vi "Configure List Step.vi"(0 "VISA resource name":refnum<visa-resource-name>, 1 "List (0: Current List)":i32(ring) items=["Current List", "Voltage List"], 2 "Execution Times (1)":i32=1, 3 "Enable List Continuously (F: Disable)":bool, 5 "Channel (1)":string="1", 7 "List Step Setting (0: Automatically)":i32(ring) items=["Automatically", "Once"], 9 "Time Point (0 sec)":dbl[](array[numeric]) format="%#_3g", 11 "error in (no error)":errorcluster, 12 "Step Value List (0.001)":dbl[](array[numeric]) format="%#_3g", 13 "Begin Trigger Signal List Step (F: Disable)":bool[](array[boolean]), 14 "End Trigger Signal List Step (F: Disable)":bool[](array[boolean])) -> (4 "VISA resource name out":refnum<visa-resource-name>, 15 "error out":errorcluster)   [LabVIEW 2020, in "Keysight E36300 Series.lvlib"]
doc: "Configures the specified list value for each list step.\n\n<b>Notes: </b>\n(1)This VI is only available on the E36312A and E36313A models.\n(2)The list is up to 100 steps.\n(3)This VI overwrites previously programmed list."
uses:
  Keysight E36300 Series.lvlib
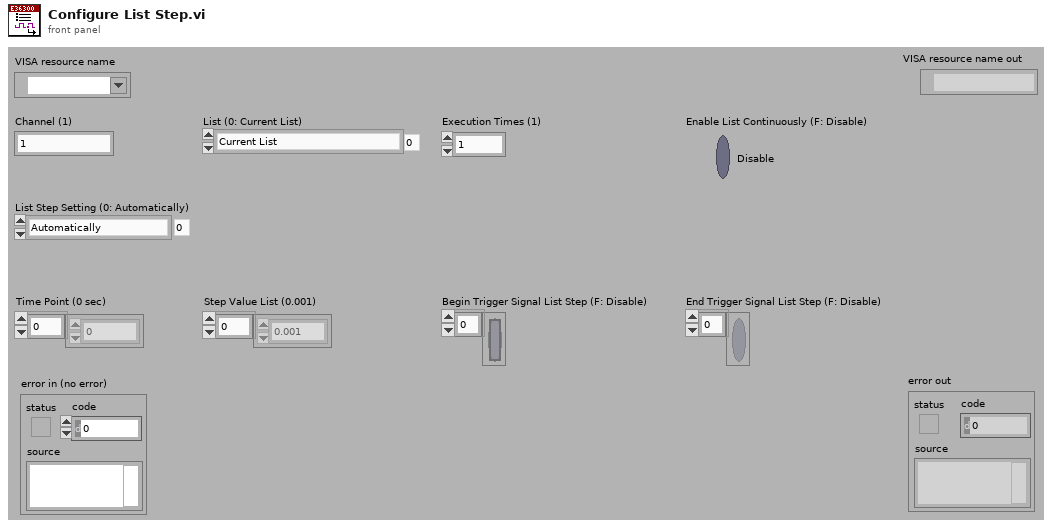
[diagram p1: front panel]
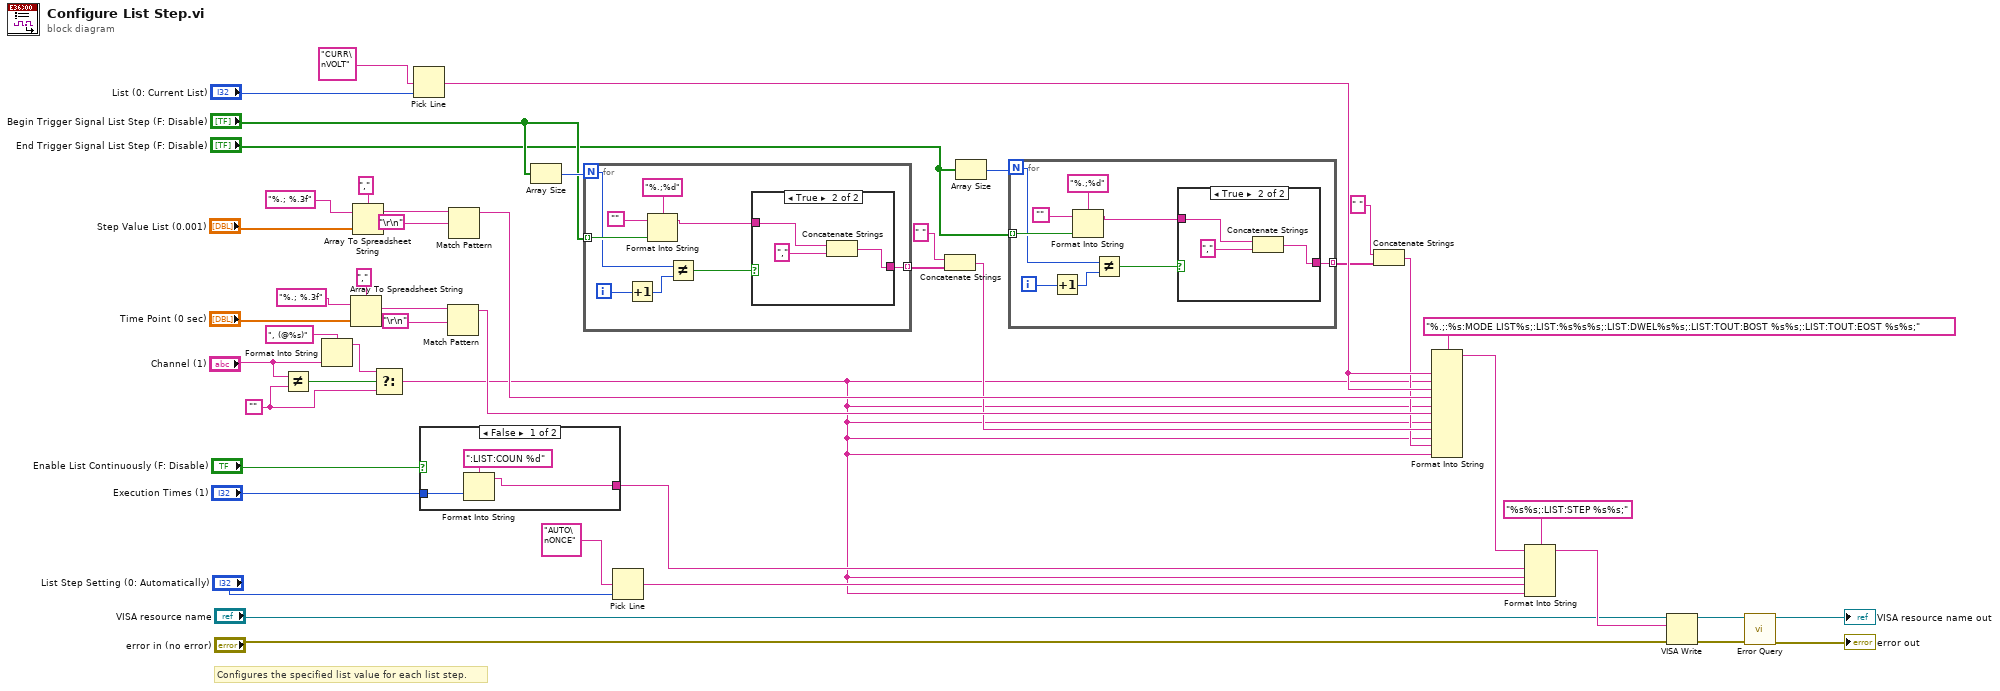
[diagram p0: block diagram]
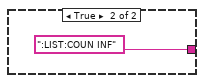
[diagram p4: hidden frame]
diagram:
  w3 = ""
  # "Configures the specified list value for each list step."
  n1 = Not Equal?(x="Channel (1)", y=w3) -> (x != y?=w4:bool)
  n2 = Format Into String(format string=", (@%s)", "Channel (1)") -> (resulting string=w5:string)  [unwired: 2 in, 1 out]
  n3 = Array To Spreadsheet String(delimiter (Tab)=",", array="Time Point (0 sec)", 3:"%.; %.3f") -> (spreadsheet string=w24:string)
  n4 = Array To Spreadsheet String(delimiter (Tab)=",", array="Step Value List (0.001)", 3:"%.; %.3f") -> (spreadsheet string=w28:string)
  n5 = Select(t=w5, s=w4, f=w3) -> (s? t:f=w1:string)
  n6 = Pick Line(multi-line string="CURR\nVOLT", line index="List (0: Current List)") -> (output string=w16:string)  [unwired: 1 in]
  n7 = case shown="False" "Enable List Continuously (F: Disable)" {
    tunnel: "Execution Times (1)" -> [w49 _]
    tunnel: [w48 ":LIST:COUN INF"] -> w22
    frame False {
      n8 = Format Into String(format string=":LIST:COUN %d", w49) -> (resulting string=w48:string)  [unwired: 2 in, 1 out]
    }
    frame True {
    }
  }
  n9 = Match Pattern(string=w24, regular expression="\r\n") -> (before substring=w15:string)  [unwired: 1 in, 3 out]
  n10 = Match Pattern(string=w28, regular expression="\r\n") -> (before substring=w27:string)  [unwired: 1 in, 3 out]
  n11 = Array Size(array="Begin Trigger Signal List Step (F: Disable)") -> (size(s)=w35:i32)
  n12 = for {
    N: w35 -> [w52]
    tunnel: [w57] -> w32 mode=indexing
    tunnel: "Begin Trigger Signal List Step (F: Disable)" -> [w53] mode=indexing
    i -> [w55]
    n13 = Increment(x=w55) -> (x+1=w56:i32)
    n14 = Format Into String(format string="%.;%d", initial string="", w53) -> (resulting string=w58:string)  [unwired: 1 in, 1 out]
    n15 = Not Equal?(x=w52, y=w56) -> (x != y?=w54:bool)
    n16 = case shown="True" w54 {
      tunnel: w58 -> [w61 w63]
      tunnel: [w61 w62] -> w57
      frame False {
      }
      frame True {
        n17 = Concatenate Strings(w63, ",") -> (w62:string)
      }
    }
  }
  n18 = Pick Line(multi-line string="AUTO\nONCE", line index="List Step Setting (0: Automatically)") -> (output string=w7:string)  [unwired: 1 in]
  n19 = Concatenate Strings(" " ("string"), w32) -> (w14:string)
  n20 = Array Size(array="End Trigger Signal List Step (F: Disable)") -> (size(s)=w13:i32)
  n21 = for {
    N: w13 -> [w65]
    tunnel: [w70] -> w11 mode=indexing
    tunnel: "End Trigger Signal List Step (F: Disable)" -> [w66] mode=indexing
    i -> [w68]
    n22 = Increment(x=w68) -> (x+1=w69:i32)
    n23 = Format Into String(format string="%.;%d", initial string="", w66) -> (resulting string=w71:string)  [unwired: 1 in, 1 out]
    n24 = Not Equal?(x=w65, y=w69) -> (x != y?=w67:bool)
    n25 = case shown="True" w67 {
      tunnel: w71 -> [w74 w76]
      tunnel: [w74 w75] -> w70
      frame False {
      }
      frame True {
        n26 = Concatenate Strings(w76, ",") -> (w75:string)
      }
    }
  }
  n27 = Concatenate Strings(" " ("string"), w11) -> (w9:string)
  n28 = Format Into String(format string="%.;:%s:MODE LIST%s;:LIST:%s%s%s;:LIST:DWEL%s%s;:LIST:TOUT:BOST %s%s;:LIST:TOUT:EOST %s%s;", w16, w1, w16, w27, w1, w15, w1, w14, w1, w9, w1) -> (resulting string=w21:string)  [unwired: 2 in, 1 out]
  n29 = Format Into String(format string="%s%s;:LIST:STEP %s%s;", initial string=w21, w22, w1, w7, w1) -> (resulting string=w20:string)  [unwired: 1 in, 1 out]
  n30 = VISA Write(VISA resource name="VISA resource name", write buffer=w20, error in (no error)="error in (no error)") -> (VISA resource name out=w44:refnum<visa-resource-name>, error out=w43:errorcluster)  [unwired: 1 out]
  n31 = call "Error Query.vi"("error in (no error)"=w43, "VISA resource name"=w44) -> ("error out"=→"error out":errorcluster, "VISA resource name out"=→"VISA resource name out":refnum<visa-resource-name>)  [unwired: 6 in, 2 out]
